vi "array_build.vi"() -> ()   [LabVIEW 2020]
panel:
  in  "Numeric 4":dbl
  in  "Numeric 3":dbl
  in  "Numeric 2":dbl
  in  "Numeric1":dbl
  out "Array":dbl[](array[numeric])
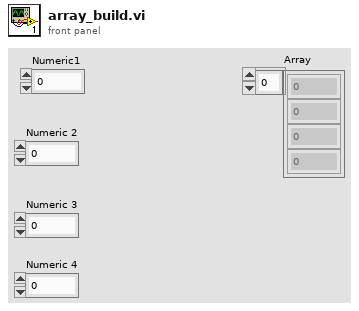
[diagram p1: front panel]
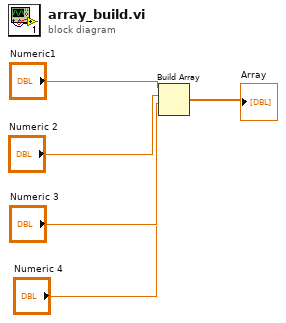
[diagram p0: block diagram]
diagram:
  n1 = Build Array("Numeric1", "Numeric 2", "Numeric 3", "Numeric 4") -> (→"Array":dbl[])
